vi "Transport.vi"(4 "Async Elements":refnum<class "Async Elements.lvclass">, 6 "VI Ref":refnum<vi>, 7 "Actor in":refnum<class "Actor.lvclass">, 10 "Refs":refnum<class "Refs.lvclass">) -> (0 "Error out":errorcluster, 5 "Actor out":refnum<class "Actor.lvclass">)   [LabVIEW 2025, in "jettl.lvlib" / "Event Transport.lvlib"]
uses:
  Event Transport.lvlib
  Actor/Actor.lvclass
  Refs/Refs.lvclass
  Async Elements/Async Elements.lvclass
  jettl.lvlib
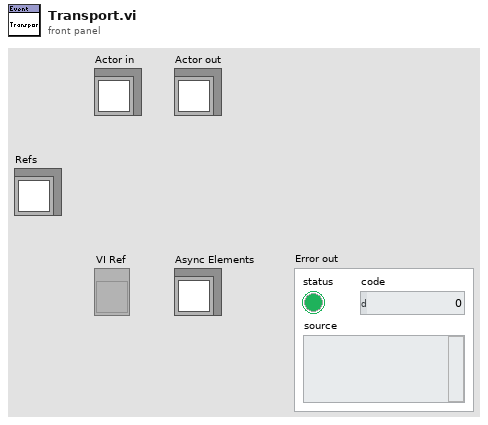
[diagram p1: front panel]
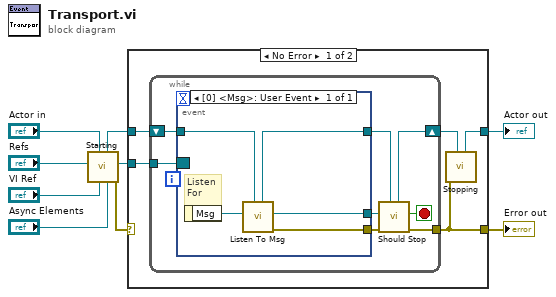
[diagram p0: block diagram]
diagram:
  n1 = call "Starting.vi"("Async Elements"="Async Elements", "VI Ref"="VI Ref", "Actor in"="Actor in", "Refs"="Refs") -> ("Error out"=w7:errorcluster, "Msg Ref"=w2:refnum<event-registration>, "Actor out"=w8:refnum<class "Actor.lvclass">)  [unwired: 5 in]
  n2 = case shown="No Error" w7 {
    selector: w7 -> [_ w28]
    tunnel: [w12 w29] -> w5
    tunnel: w8 -> [w11 w29]
    tunnel: [w14 w28] -> w9
    tunnel: w2 -> [w10 _]
    frame No Error {
      n3 = while {
        shift-right: [w17] -> w13
        shift-left: w11 -> [w22]
        tunnel: [w20] -> w14
        tunnel: w10 -> [w15]
        stop <- w19 stop-if-true
        n4 = event shown="[0] <Msg>: User Event" {
          selector: w15 -> [_]
          dyn-events: _ -> [_]
          timeout: _ -> [_]
          tunnel: w22 -> [w27]
          tunnel: [w25] -> w16
          tunnel: [w24] -> w21
          tunnel: [w23] -> w18
          event User Event {
            # "Listen\nFor"
            n5 = event-data() -> ("Msg"=w26:refnum<class "Msg.lvclass">)  [unwired: 1 in]
            n6 = call "Listen To Msg.vi"("Actor in"=w27, "Msg"=w26) -> ("Error out"=w24:errorcluster, "Msg Output"=w23:refnum<class "Msg Output.lvclass">, "Actor out"=w25:refnum<class "Actor.lvclass">)  [unwired: 7 in]
          }
        }
        n7 = call "Should Stop.vi"("Actor in"=w16, "Error in"=w21, "Msg Output"=w18) -> ("Error out"=w20:errorcluster, "Stop"=w19:bool, "Actor out"=w17:refnum<class "Actor.lvclass">)  [unwired: 6 in]
      }
      n8 = call "Stopping.vi"("Actor in"=w13, "Error in"=w14) -> ("Actor out"=w12:refnum<class "Actor.lvclass">)  [unwired: 9 in]
    }
    frame Error {
    }
  }
  "Error out" <- w9
  "Actor out" <- w5
